vi "U3 Thermocouple Example.vi"(8 "error in":errorcluster) -> (0 "error out":errorcluster)   [LabVIEW 2021]
panel:
  in  "Gain":dbl=51.0 format="%.4f"
  in  "Cold Junction Sensor Offset [degK]":dbl format="%.4f"
  in  "Cold Junction Sensor Slope [degK/V]":dbl=1.0 format="%.4f"
  in  "Cold Junction Sensor Channel":i32=30
  out "Temperatures (Deg C)":dbl[](array[numeric]) format="%.2f"
  out "Cold Junction\nTemperature (Deg C)":dbl format="%.2f"
  in  "Offset Voltages":dbl[](array[numeric])=[0.0, 0.0] format="%.6f"
  in  "Channels":i32[](array[numeric])=[4, 5]
  out "Raw Readings":dbl[](array[numeric]) format="%.6f"
  out "Error Message":string
  # "Uses the first found U3 over USB.  Requires UD driver V2.60+.\n\nAquires multiple analog input channels and performs a K type thermocouple conversion on them.  For\nimproved accuracy, set the TCs near the U3 so they are at the same ambient temperature and thus\nthe measured voltage should be zero.  With the U3 powered-up, allow 20 minutes for everything\nto stabilize.  Then note the voltage offset in the \"Readings\" array, and enter this in the \"Offset\" array."
  # "If using an LJTIA (or other amplifier) to amplify the\nthermocouple voltages, enter the gain here."
  # "The voltage from a thermocouple corresponds to the temperature\ndifference between one end and the other.  To determine the temp\nat the remote end, we must know the temperature at the local end.\nThe local end is called the cold junction, and in this case is\nthe U3/LJTIA.  Enter the channel # from which to read the cold\njuntion temperature, and enter the slope/offset required to convert\nthat temperature to degrees K."
  # "Internal Sensor = 30"
  # "Internal=1, EI-1022=100, EI-1034=55.56"
  # "Internal=0, EI-1022=0, EI-1034=255.37"
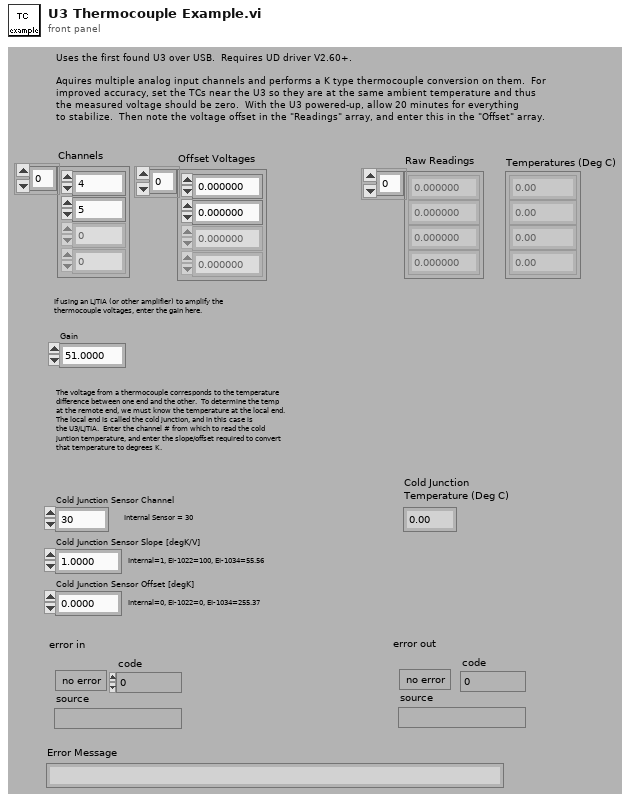
[diagram p1: front panel]
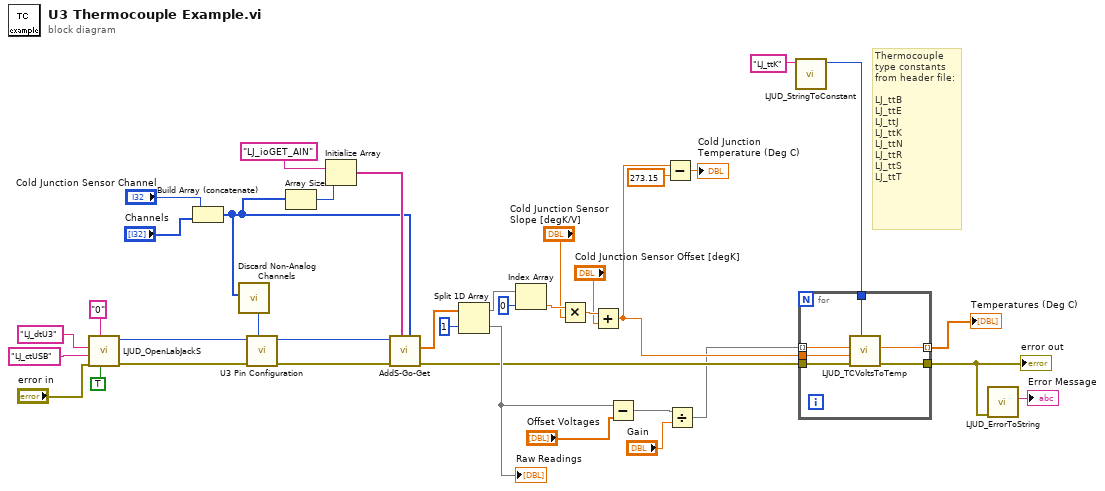
[diagram p0: block diagram]
diagram:
  # "Thermocouple\ntype constants\nfrom header file:\n\nLJ_ttB\nLJ_ttE\nLJ_ttJ\nLJ_ttK\nLJ_ttN\nLJ_ttR\nLJ_ttS\nLJ_ttT"
  n1 = call "LJUD_OpenLabJackS.vi"("FirstFound"=TRUE, "Address"="0", "error in"="error in", "ConnectionType"="LJ_ctUSB", "DeviceType"="LJ_dtU3") -> ("error out"=w9:errorcluster, "Handle"=w6:i32)  [unwired: 4 in, 1 out]
  n2 = Build Array (concatenate)("Cold Junction Sensor Channel", "Channels") -> (w1:i32[])
  n3 = call "Discard Non-Analog Channels.vi"("Channels In"=w1) -> ("FIO/EIO Analog Enable"=w3:i32)  [unwired: 7 in, 3 out]
  n4 = call "U3 Pin Configuration.vi"("FIO/EIO Analog Enable"=w3, "error in"=w9, "Handle In"=w6) -> ("error out"=w8:errorcluster, "Handle Out"=w7:i32)  [unwired: 7 in]
  n5 = Array Size(array=w1) -> (size(s)=w4:i32)
  n6 = Initialize Array("LJ_ioGET_AIN" ("IOType"), w4) -> (w33:string[])
  n7 = call "AddS-Go-Get.vi"("Channels"=w1, "IOTypes"=w33, "error in"=w8, "Handle In"=w7) -> ("error out"=w15:errorcluster, "Values Read"=w28:dbl[])  [unwired: 5 in, 1 out]
  n8 = Split 1D Array(array=w28, index=1) -> (first subarray=w27:dbl[], second subarray=w16:dbl[])
  "Raw Readings" <- w16
  n9 = Index Array(array=w27, index=0 ("Index")) -> (element=w25:dbl)
  n10 = Multiply(x=w25, y="Cold Junction Sensor Slope [degK/V]") -> (x*y=w24:dbl)
  n11 = Add(x=w24, y="Cold Junction Sensor Offset [degK]") -> (x+y=w14:dbl)
  n12 = Subtract(x=w16, y="Offset Voltages") -> (x-y=w17:dbl[])
  n13 = Subtract(x=w14, y=273.15) -> (x-y=→"Cold Junction\nTemperature (Deg C)":dbl)
  n14 = Divide(x=w17, y="Gain") -> (x/y=w13:dbl[])
  n15 = call "LJUD_StringToConstant.vi"("String"="LJ_ttK") -> ("Constant Number"=w12:i32)  [unwired: 9 in, 1 out]
  n16 = for {
    tunnel: w15 -> [w44]
    tunnel: w14 -> [w43]
    tunnel: w13 -> [w42] mode=indexing
    tunnel: w12 -> [w41]
    tunnel: [w40] -> w11
    tunnel: [w39] -> w10 mode=indexing
    n17 = call "LJUD_TCVoltsToTemp.vi"("TCType"=w41, "error in"=w44, "CJTempK"=w43, "TCVolts"=w42) -> ("error out"=w40:errorcluster, "TCTempC"=w39:dbl)  [unwired: 4 in, 2 out]
  }
  "error out" <- w11
  "Temperatures (Deg C)" <- w10
  n18 = call "LJUD_ErrorToString.vi"("error in"=w11) -> ("String"=→"Error Message":string)  [unwired: 10 in]
